vi "getReturn_Number_Int32.vi"(8 "error in (no error)":errorcluster, 9 "return list in":T1[](array[typedef]), 11 "LabVIEW-Python-Interface in":refnum<class "PyLVi.lvclass">) -> (0 "error out":errorcluster, 1 "return list out":T1[](array[typedef]), 2 "data out":i32, 3 "LabVIEW-Python-Interface out":refnum<class "PyLVi.lvclass">)   [LabVIEW 2016, in "PyLVi.lvlib" / "PyLVi.lvclass"]
uses:
  PyLVi.lvclass
  Controls/ArgumentStructure.ctl
  Controls/DescriptorStructure.ctl
  Controls/ArgumentType.ctl
  Controls/DataType.ctl
panel:
  out "data string":string
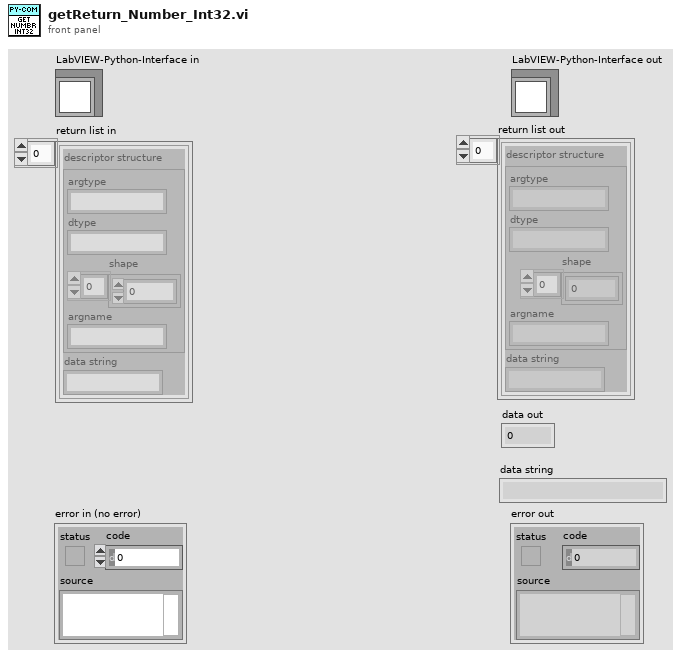
[diagram p1: front panel]
types:
  T1 = typedef "PyLVi.lvlib/PyLVi.lvclass/ArgumentStructure.ctl" = cluster{"descriptor structure":T2, "data string":string}
  T2 = typedef "PyLVi.lvlib/PyLVi.lvclass/DescriptorStructure.ctl" = cluster{"argtype":string, "dtype":string, "shape":u32[], "argname":string}
  T3 = enum16{"big-endian, network order", "native, host order", "little-endian"}
  T4 = typedef "PyLVi.lvlib/PyLVi.lvclass/DataType.ctl" = enum16{"bool", "string", "int16", "int32", "float32", "float64", "complex128"}
  T5 = typedef "PyLVi.lvlib/PyLVi.lvclass/ArgumentType.ctl" = enum8{"bool", "numeric", "string", "dict", "ndarray", "ndarray2d"}
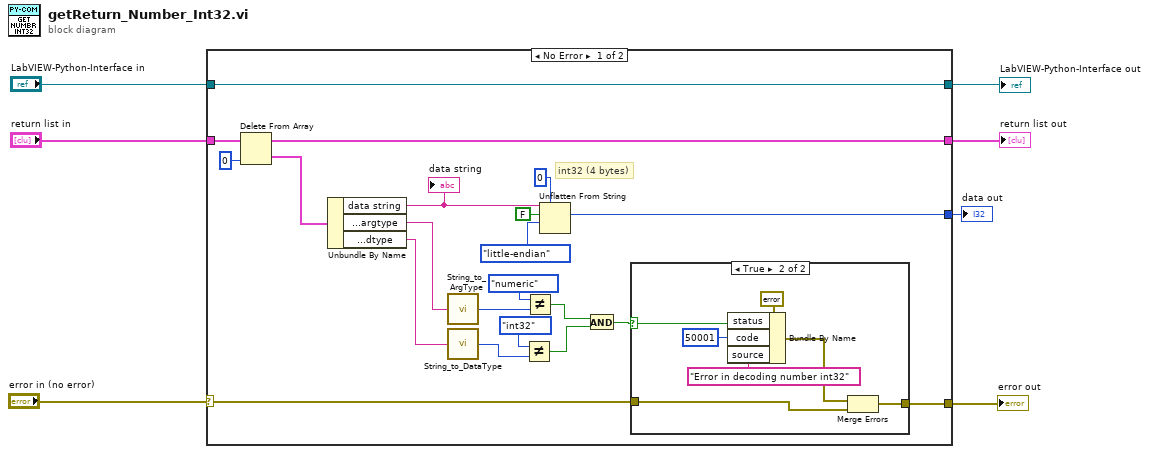
[diagram p0: block diagram]
diagram:
  n1 = case shown="No Error" "error in (no error)" {
    selector: "error in (no error)" -> [w11 w38]
    tunnel: [w19 w38] -> w2
    tunnel: [w13 w39] -> w5
    tunnel: "LabVIEW-Python-Interface in" -> [w13 w39]
    tunnel: "return list in" -> [w21 w37]
    tunnel: [w20 w37] -> w4
    tunnel: [w9 _] -> w1
    frame No Error {
      # "int32 (4 bytes)"
      n2 = Delete From Array(array=w21, index=0) -> (deleted portion=w22:T1, array with subset deleted=w20:T1[])  [unwired: 1 in]
      n3 = Unbundle By Name(w22) -> ("data string"=w14:string, "descriptor structure.argtype"=w18:string, "descriptor structure.dtype"=w17:string)
      "data string" <- w14
      n4 = call "String_to_ArgType.vi"("arg type string"=w18) -> ("arg type"=w23:T5)  [unwired: 4 in]
      n5 = call "String_to_DataType.vi"("data type string"=w17) -> ("data type"=w25:T4)  [unwired: 4 in]
      n6 = Not Equal?(x=DataType."int32", y=w25) -> (x != y?=w28:bool)
      n7 = Not Equal?(x=ArgumentType."numeric", y=w23) -> (x != y?=w27:bool)
      n8 = Unflatten From String(type=0, binary string=w14, data includes array or string size? (T)=FALSE, byte order (0:big-endian, network order)=T3."little-endian") -> (value=w9:i32)  [unwired: 1 in, 2 out]
      n9 = And(x=w27, y=w28) -> (x .and. y?=w12:bool)
      n10 = case shown="True" w12 {
        selector: w12 -> [_ w33]
        tunnel: [w29 w32] -> w19
        tunnel: w11 -> [w29 w30]
        frame False {
        }
        frame True {
          n11 = Bundle By Name(cluster=errorcluster {"status"=FALSE, "code"=0, "source"=""} ("error constant"), "status"=w33, "code"=50001, "source"="Error in decoding number int32") -> (w31:errorcluster)
          n12 = Merge Errors(w31, w30) -> (w32:errorcluster)
        }
      }
    }
    frame Error {
    }
  }
  "error out" <- w2
  "LabVIEW-Python-Interface out" <- w5
  "return list out" <- w4
  "data out" <- w1
